vi "LJM_eWriteNames.vi"(0 "Handle In":i32, 1 "NumFrames (Auto-Detect)":i32=-1, 5 "aNames":string[](array[string]), 9 "aValuesIn":dbl[](array[numeric]) format="%.2f", 11 "error in":errorcluster) -> (4 "Handle Out":i32, 14 "ErrorAddress":i32, 15 "error out":errorcluster)   [LabVIEW 2025]
panel:
  # "1/20/2015:  Default value of NumFrames changed to -1 which\nequates to Auto-Detect.  If NumFrames = -1, then the NumFrames\ncontrol is ignored and the size of aNames/aAddresses is used to\ndetermine how many frames there are."
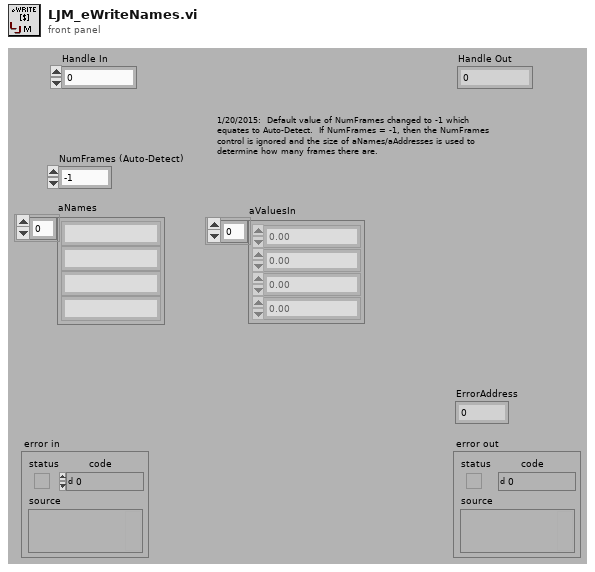
[diagram p1: front panel]
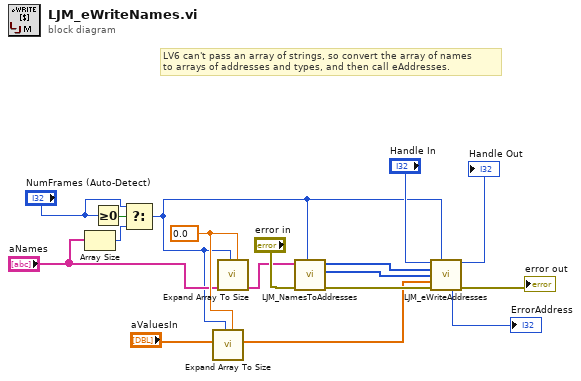
[diagram p0: block diagram]
diagram:
  w16 = 0.0 ("Default Value")
  # "LV6 can't pass an array of strings, so convert the array of names\nto arrays of addresses and types, and then call eAddresses."
  n1 = Array Size(array="aNames") -> (size(s)=w3:i32)
  n2 = Greater Or Equal To 0?(x="NumFrames (Auto-Detect)") -> (x >= 0?=w5:bool)
  n3 = Select(t="NumFrames (Auto-Detect)", s=w5, f=w3) -> (s? t:f=w1:i32)
  n4 = call "Expand Array To Size.vi"("Default Value"=w16, "# Elements"=w1, "DBL Array In"="aValuesIn") -> ("DBL Array Out"=w6:dbl[])  [unwired: 4 in, 4 out]
  n5 = call "Expand Array To Size.vi"("Default Value"=w16, "# Elements"=w1, "String Array In"="aNames") -> ("String Array Out"=w14:string[])  [unwired: 4 in, 4 out]
  n6 = call "LJM_NamesToAddresses.vi"("NumFrames (Auto-Detect)"=w1, "error in"="error in", "aNames"=w14) -> ("error out"=w13:errorcluster, "aTypes"=w7:i32[], "aAddresses"=w8:i32[])  [unwired: 6 in]
  n7 = call "LJM_eWriteAddresses.vi"("Handle In"="Handle In", "NumFrames (Auto-Detect)"=w1, "aAddresses"=w8, "aTypes"=w7, "aValues"=w6, "error in"=w13) -> ("Handle Out"=→"Handle Out":i32, "ErrorAddress"=→"ErrorAddress":i32, "error out"=→"error out":errorcluster)  [unwired: 7 in]
